vi "Start.vi"(8 "error in (no error)":errorcluster, 9 "Channel Data (DBLs Only)":T1, 10 "Real-Time System Data":T2, 11 "Configuration Data":T3) -> (0 "error out":errorcluster, 1 "Channel Data (DBLs Only)":T1, 2 "Real-Time System Data":T2, 3 "Configuration Data":T3)   [LabVIEW 2010]
uses:
  Configuration Data.ctl
  Real-Time System Data.ctl
  Channel Data.ctl
panel:
  # "Controls"
  # "Indicators"
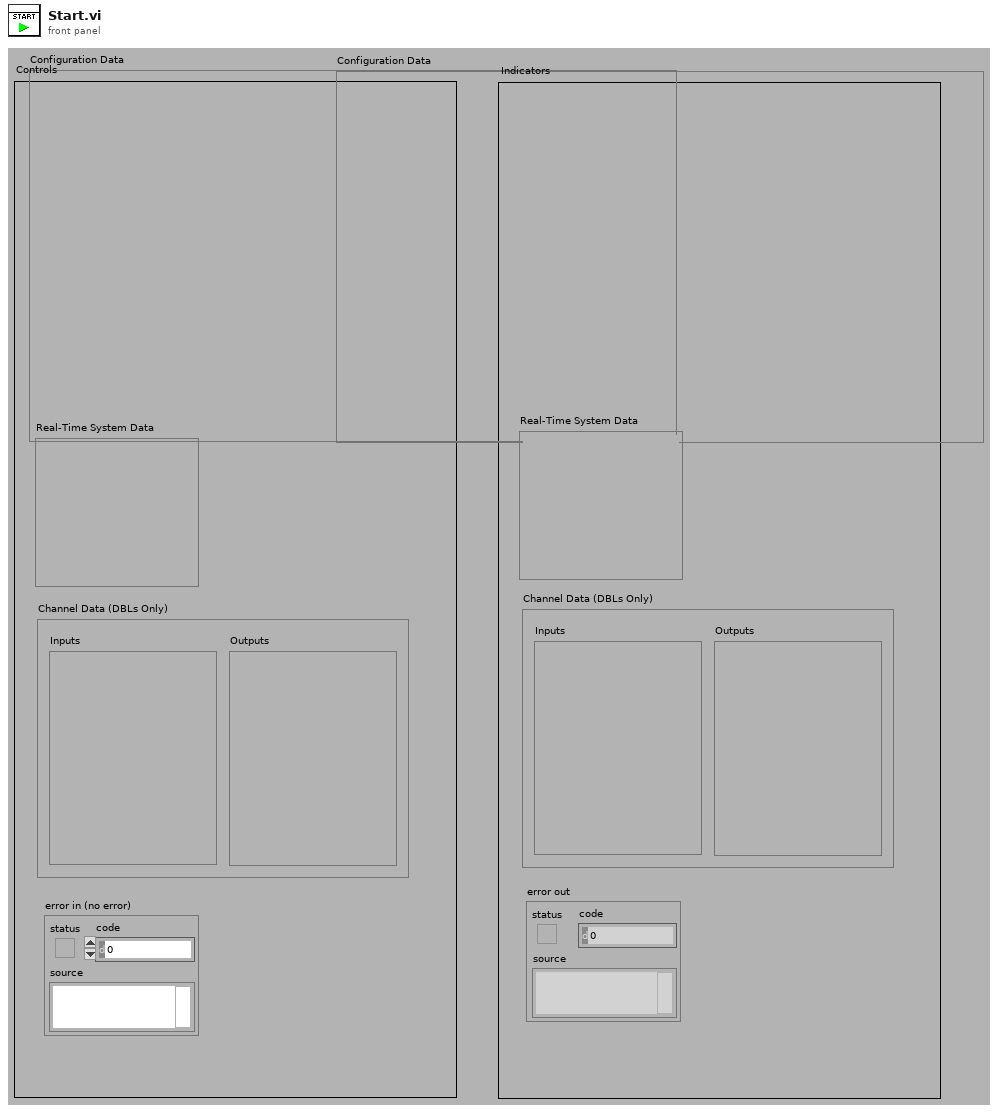
[diagram p1: front panel]
types:
  T1 = typedef "Channel Data.ctl" = cluster{"Inputs":cluster{}, "Outputs":cluster{}}
  T2 = typedef "Real-Time System Data.ctl" = cluster{}
  T3 = typedef "Configuration Data.ctl" = cluster{}
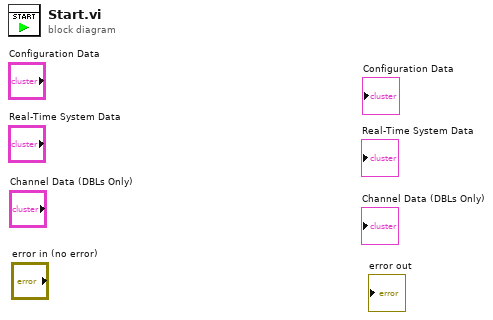
[diagram p0: block diagram]
diagram:
